vi "WT210 Get Data.vi"(6 "Collect Element 3 Data":bool, 8 "error in (no error)":errorcluster, 10 "Uthd:Element 1":dbl format="%#_13g", 11 "VISA resource name":refnum<visa-resource-name>) -> (0 "error out":errorcluster, 1 "Power":sgl caption="Measure Value" format="%.3f", 2 "VISA resource name out":refnum<visa-resource-name>, 3 "Power Data":T1={"Current (A):Element 1"=236.2, "Current (A):Element 2"=17.749, "Power (W):Sigma"=4192.0, "Watt Hours (Wh):Sigma"=0.0, "Voltage (V):Element 2"=236.2, "Voltage (V):Element 1"=236.2, "Current Crest Factor:Element 1"=0.0, "Current Crest Factor:Element 2"=0.0, "Voltage Harmonic (%):Element 1"=0.0, "Voltage Harmonic (%):Element 2"=0.0, "Voltage Crest Factor:Element 1"=0.0, "Voltage Crest Factor:Element 2"=0.0, "Time:Element 1"=0.0, "Frequency (Hz):Element 1"=0.0, "Apparent Power (VA):Element 1"=0.0, "Apparent Power (VA):Element 2"=0.0, "Power Factor:Element 1"=0.0, "Power Factor:Element 2"=0.0, "Max Watt Hours"=0.0, "Voltage (V):Element 2 Avg"=0.0, "Voltage (V):Element 1 Avg"=0.0} {"Voltage (V):Element 1 Avg" format="%.3g"; "Voltage (V):Element 2 Avg" format="%.3g"; "Max Watt Hours" format="%.3g"; "Power Factor:Element 2" format="%.3g"; "Power Factor:Element 1" format="%.3g"; "Apparent Power (VA):Element 2" format="%.3g"; "Apparent Power (VA):Element 1" format="%.3g"; "Frequency (Hz):Element 1" format="%.3g"; "Time:Element 1" format="%.3g"; "Voltage Crest Factor:Element 2" format="%.3g"; "Voltage Crest Factor:Element 1" format="%.3g"; "Voltage Harmonic (%):Element 2" format="%.3g"; "Voltage Harmonic (%):Element 1" format="%.3g"; "Current Crest Factor:Element 2" format="%.3g"; "Current Crest Factor:Element 1" format="%.3g"; "Voltage (V):Element 1" format="%.3g"; "Voltage (V):Element 2" format="%.3g"; "Watt Hours (Wh):Sigma" format="%.3f"; "Power (W):Sigma" format="%.3g"; "Current (A):Element 2" format="%.3g"; "Current (A):Element 1" format="%.3g"}, 5 "Yokogawa Data":string[][](array[string]), 7 "Yokogawa DBL Array":dbl[](array[numeric]))   [LabVIEW 2016]
uses:
  Trunk/Utility/Type Definitions/UTILITY Power Data.ctl
panel:
  in  "Uthd:Element 2":dbl format="%#_13g"
  in  "Dryer PowerData":T1={"Current (A):Element 1"=236.2, "Current (A):Element 2"=17.749, "Power (W):Sigma"=4192.0, "Watt Hours (Wh):Sigma"=0.0, "Voltage (V):Element 2"=236.2, "Voltage (V):Element 1"=236.2, "Current Crest Factor:Element 1"=0.0, "Current Crest Factor:Element 2"=0.0, "Voltage Harmonic (%):Element 1"=0.0, "Voltage Harmonic (%):Element 2"=0.0, "Voltage Crest Factor:Element 1"=0.0, "Voltage Crest Factor:Element 2"=0.0, "Time:Element 1"=0.0, "Frequency (Hz):Element 1"=0.0, "Apparent Power (VA):Element 1"=0.0, "Apparent Power (VA):Element 2"=0.0, "Power Factor:Element 1"=0.0, "Power Factor:Element 2"=0.0, "Max Watt Hours"=0.0, "Voltage (V):Element 2 Avg"=0.0, "Voltage (V):Element 1 Avg"=0.0} {"Voltage (V):Element 1 Avg" format="%.3g"; "Voltage (V):Element 2 Avg" format="%.3g"; "Max Watt Hours" format="%.3g"; "Power Factor:Element 2" format="%.3g"; "Power Factor:Element 1" format="%.3g"; "Apparent Power (VA):Element 2" format="%.3g"; "Apparent Power (VA):Element 1" format="%.3g"; "Frequency (Hz):Element 1" format="%.3g"; "Time:Element 1" format="%.3g"; "Voltage Crest Factor:Element 2" format="%.3g"; "Voltage Crest Factor:Element 1" format="%.3g"; "Voltage Harmonic (%):Element 2" format="%.3g"; "Voltage Harmonic (%):Element 1" format="%.3g"; "Current Crest Factor:Element 2" format="%.3g"; "Current Crest Factor:Element 1" format="%.3g"; "Voltage (V):Element 1" format="%.3g"; "Voltage (V):Element 2" format="%.3g"; "Watt Hours (Wh):Sigma" format="%.3f"; "Power (W):Sigma" format="%.3g"; "Current (A):Element 2" format="%.3g"; "Current (A):Element 1" format="%.3g"}
  # "Output Data from WT210"
  # "Wh"
  # "V"
  # "A"
  # "V Hz"
  # "W"
  # "PF"
  # "VA"
  # "V CF"
  # "WT210 can only take one harmonic reading"
  # "A CF"
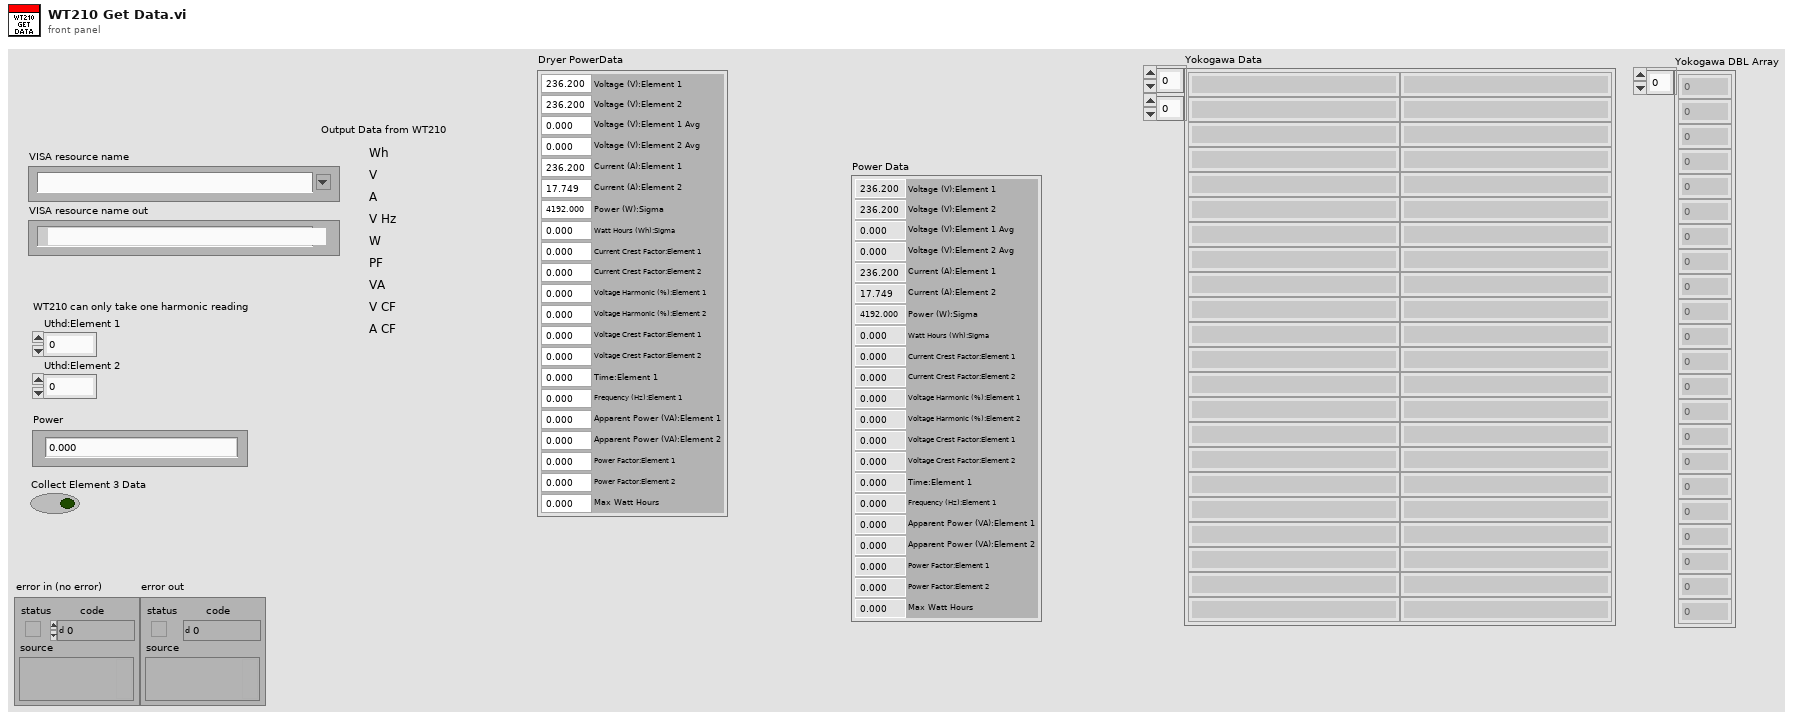
[diagram p1: front panel]
types:
  T1 = typedef "UTILITY Power Data.ctl" = cluster{"Current (A):Element 1":dbl, "Current (A):Element 2":dbl, "Power (W):Sigma":dbl, "Watt Hours (Wh):Sigma":dbl, "Voltage (V):Element 2":dbl, "Voltage (V):Element 1":dbl, "Current Crest Factor:Element 1":dbl, "Current Crest Factor:Element 2":dbl, "Voltage Harmonic (%):Element 1":dbl, "Voltage Harmonic (%):Element 2":dbl, "Voltage Crest Factor:Element 1":dbl, "Voltage Crest Factor:Element 2":dbl, "Time:Element 1":dbl, "Frequency (Hz):Element 1":dbl, "Apparent Power (VA):Element 1":dbl, "Apparent Power (VA):Element 2":dbl, "Power Factor:Element 1":dbl, "Power Factor:Element 2":dbl, "Max Watt Hours":dbl, "Voltage (V):Element 2 Avg":dbl, "Voltage (V):Element 1 Avg":dbl}
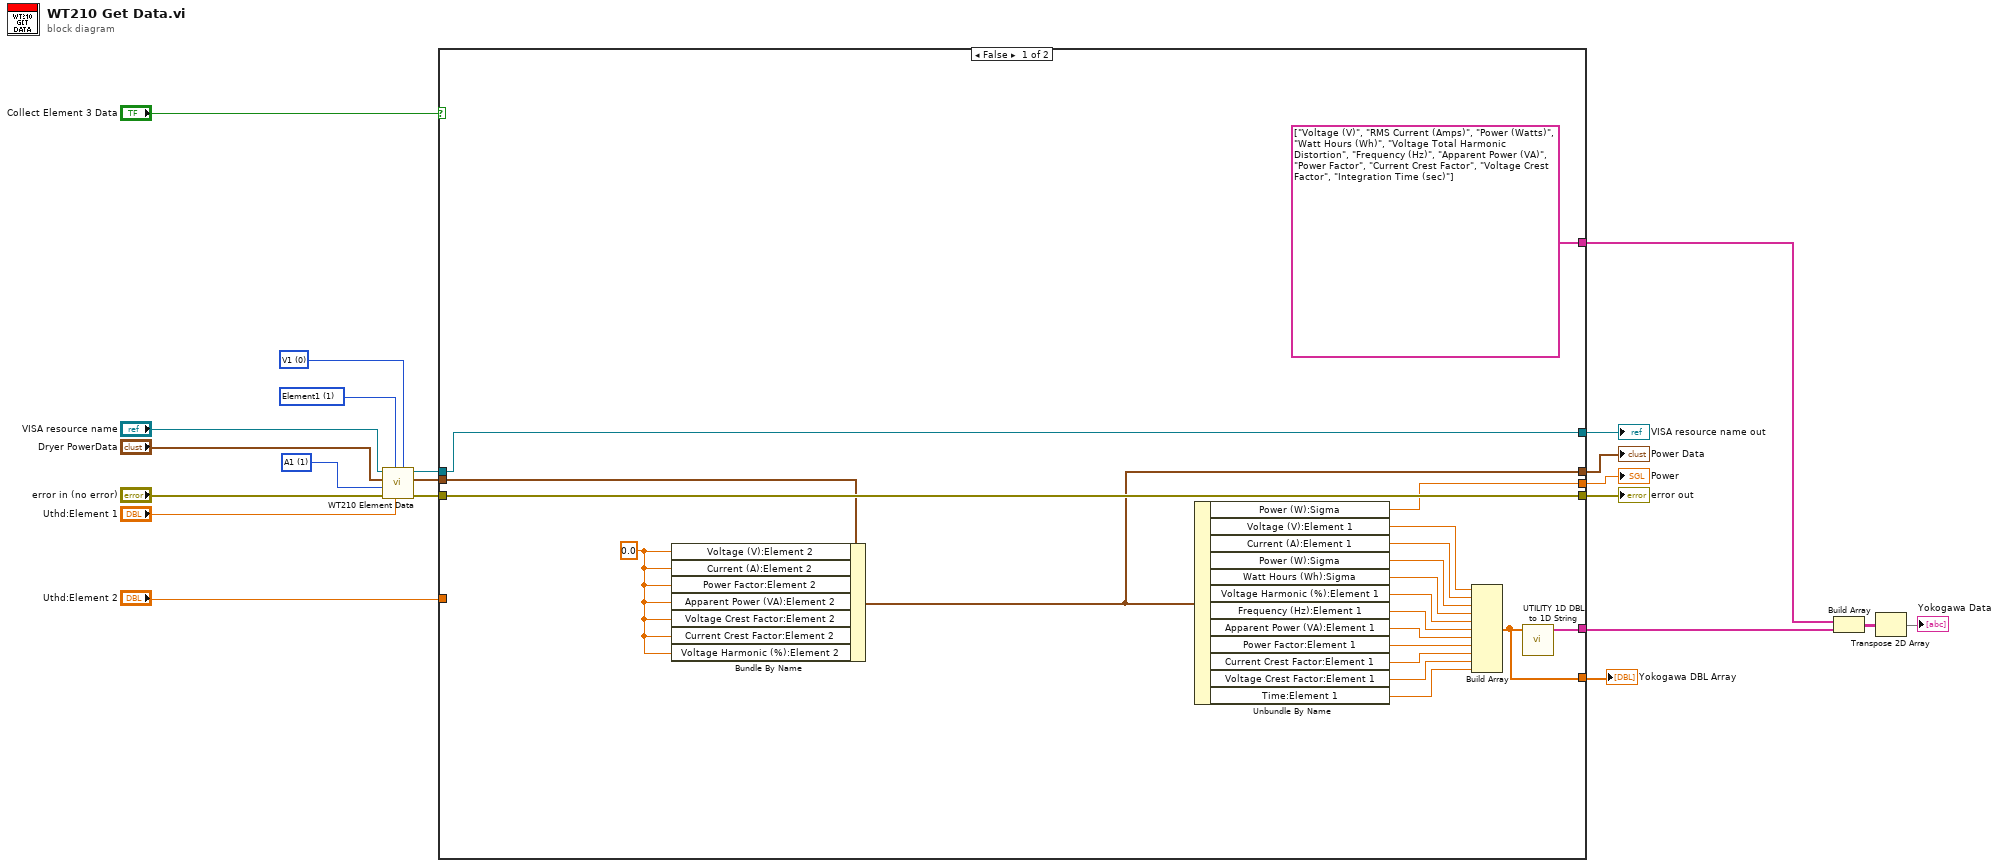
[diagram p0: block diagram]
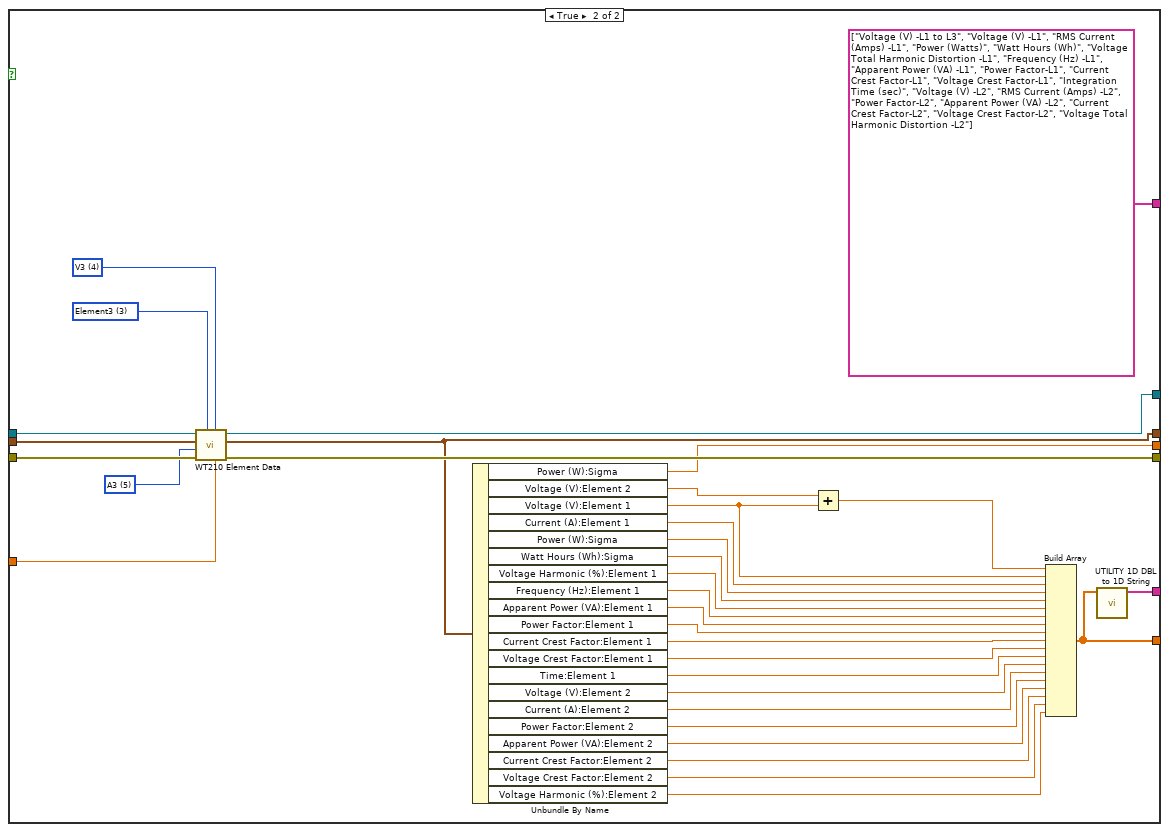
[diagram p2: hidden frame]
diagram:
  w16 = u16 1 items=["", "Element1", "Element2", "Element3", "Sigma"] ("Element (1: Element 1)")
  w18 = u16 1 items=["V1", "A1", "V2", "A2", "V3", "A3"] ("C Factor (0: V)")
  w8 = u16 0 items=["V1", "A1", "V2", "A2", "V3", "A3"] ("C Factor (0: V)")
  n1 = call "WT210 Element Data.vi"("C Factor (0: V) 2"=w8, "Uthd:Element 1"="Uthd:Element 1", "Element (1: Element 1)"=w16, "error in (no error)"="error in (no error)", "C Factor (0: V)"=w18, "Dryer PowerData in"="Dryer PowerData", "VISA Refnum in"="VISA resource name") -> ("error out"=w15:errorcluster, "Dryer PowerData out"=w10:T1, "VISA Refnum out"=w14:refnum<visa-resource-name>)  [unwired: 2 in]
  n2 = case shown="False" "Collect Element 3 Data" {
    tunnel: w15 -> [w41 w75]
    tunnel: w14 -> [w40 w74]
    tunnel: [w40 w73] -> w13
    tunnel: [w41 w72] -> w12
    tunnel: w10 -> [w39 w71]
    tunnel: [w24 w57] -> w9
    tunnel: "Uthd:Element 2" -> [_ w68]
    tunnel: [string[] ["Voltage (V)", "RMS Current (Amps)", "Power (Watts)", "Watt Hours (Wh)", "Voltage Total Harmonic Distortion", "Frequency (Hz)", "Apparent Power (VA)", "Power Factor", "Current Crest Factor", "Voltage Crest Factor", "Integration Time (sec)"] string[] ["Voltage (V) -L1 to L3", "Voltage (V) -L1", "RMS Current (Amps) -L1", "Power (Watts)", "Watt Hours (Wh)", "Voltage Total Harmonic Distortion -L1", "Frequency (Hz) -L1", "Apparent Power (VA) -L1", "Power Factor-L1", "Current Crest Factor-L1", "Voltage Crest Factor-L1", "Integration Time (sec)", "Voltage (V) -L2", "RMS Current (Amps) -L2", "Power Factor-L2", "Apparent Power (VA) -L2", "Current Crest Factor-L2", "Voltage Crest Factor-L2", "Voltage Total Harmonic Distortion -L2"]] -> w5
    tunnel: [w25 w48] -> w4
    tunnel: [w23 w49] -> w3
    tunnel: [w22 w47] -> w2
    frame False {
      w38 = 0.0 ("Uthd:Element 2")
      n3 = Bundle By Name(cluster=w39, "Voltage (V):Element 2"=w38, "Current (A):Element 2"=w38, "Power Factor:Element 2"=w38, "Apparent Power (VA):Element 2"=w38, "Voltage Crest Factor:Element 2"=w38, "Current Crest Factor:Element 2"=w38, "Voltage Harmonic (%):Element 2"=w38) -> (w24:T1)
      n4 = Unbundle By Name(w24) -> ("Power (W):Sigma"=w22:dbl, "Voltage (V):Element 1"=w27:dbl, "Current (A):Element 1"=w28:dbl, "Power (W):Sigma"=w37:dbl, "Watt Hours (Wh):Sigma"=w29:dbl, "Voltage Harmonic (%):Element 1"=w30:dbl, "Frequency (Hz):Element 1"=w31:dbl, "Apparent Power (VA):Element 1"=w32:dbl, "Power Factor:Element 1"=w33:dbl, "Current Crest Factor:Element 1"=w34:dbl, "Voltage Crest Factor:Element 1"=w35:dbl, "Time:Element 1"=w36:dbl)
      n5 = Build Array(w27, w28, w37, w29, w30, w31, w32, w33, w34, w35, w36) -> (w23:dbl[])
      n6 = call "UTILITY 1D DBL to 1D String.vi"("1D DBL"=w23) -> ("1D String"=w25:string[])  [unwired: 10 in]
    }
    frame True {
      w45 = u16 4 items=["V1", "A1", "V2", "A2", "V3", "A3"] ("C Factor (0: V)")
      w69 = u16 5 items=["V1", "A1", "V2", "A2", "V3", "A3"] ("C Factor (0: V)")
      w70 = u16 3 items=["", "Element1", "Element2", "Element3", "Sigma"] ("Element (1: Element 1)")
      n7 = call "WT210 Element Data.vi"("Uthd:Element 2"=w68, "C Factor (0: V) 2"=w45, "Element (1: Element 1)"=w70, "error in (no error)"=w75, "C Factor (0: V)"=w69, "Dryer PowerData in"=w71, "VISA Refnum in"=w74) -> ("error out"=w72:errorcluster, "Dryer PowerData out"=w57:T1, "VISA Refnum out"=w73:refnum<visa-resource-name>)  [unwired: 2 in]
      n8 = Unbundle By Name(w57) -> ("Power (W):Sigma"=w47:dbl, "Voltage (V):Element 2"=w42:dbl, "Voltage (V):Element 1"=w43:dbl, "Current (A):Element 1"=w58:dbl, "Power (W):Sigma"=w67:dbl, "Watt Hours (Wh):Sigma"=w59:dbl, "Voltage Harmonic (%):Element 1"=w60:dbl, "Frequency (Hz):Element 1"=w61:dbl, "Apparent Power (VA):Element 1"=w62:dbl, "Power Factor:Element 1"=w63:dbl, "Current Crest Factor:Element 1"=w64:dbl, "Voltage Crest Factor:Element 1"=w65:dbl, "Time:Element 1"=w66:dbl, "Voltage (V):Element 2"=w56:dbl, "Current (A):Element 2"=w55:dbl, "Power Factor:Element 2"=w54:dbl, "Apparent Power (VA):Element 2"=w53:dbl, "Current Crest Factor:Element 2"=w52:dbl, "Voltage Crest Factor:Element 2"=w51:dbl, "Voltage Harmonic (%):Element 2"=w50:dbl)
      n9 = Add(x=w42, y=w43) -> (x+y=w44:dbl)
      n10 = Build Array(w44, w43, w58, w67, w59, w60, w61, w62, w63, w64, w65, w66, w56, w55, w54, w53, w52, w51, w50) -> (w49:dbl[])
      n11 = call "UTILITY 1D DBL to 1D String.vi"("1D DBL"=w49) -> ("1D String"=w48:string[])  [unwired: 10 in]
    }
  }
  "Power Data" <- w9
  "VISA resource name out" <- w13
  "error out" <- w12
  "Yokogawa DBL Array" <- w3
  "Power" <- w2
  n12 = Build Array(w5, w4) -> (w17:string[][])
  n13 = Transpose 2D Array(2D array=w17) -> (transposed array=→"Yokogawa Data":string[][])
